vi "vision_webcam_V2.vi"(11 "dup Message Queue 2":refnum<queue>) -> ()   [LabVIEW 2017]
uses:
  UI Error Handlers/support/Message Queue/Message Cluster.ctl
  <vilib>/vision/Image Controls.llb/IMAQ Image.ctl
  camera_array_1.ctl
  <vilib>/userdefined/High Color/IMAQdx.ctl
  <vilib>/vision/Avi.llb/IMAQ AVI2 Refnum.ctl
  <vilib>/vision/Avi.llb/IMAQ AVI2 Codec Path.ctl
  Globals/Global - All RT Loop Stop.vi
  Globals/Global - Configuration Options.vi
  <vilib>/vision/driver/NI_Vision_Acquisition_Software.lvlib
  UI Error Handlers/support/Message Queue/Message Queue.lvlib
panel:
  out "Images":T1
  out "Array":T2[](array[typedef])
  out "Webcam":T2(plugin-control)
  out "Codec Names 2":string[](array[string])
  out "concatenated string 4":string
  out "error out":errorcluster
  out "x-y":u32
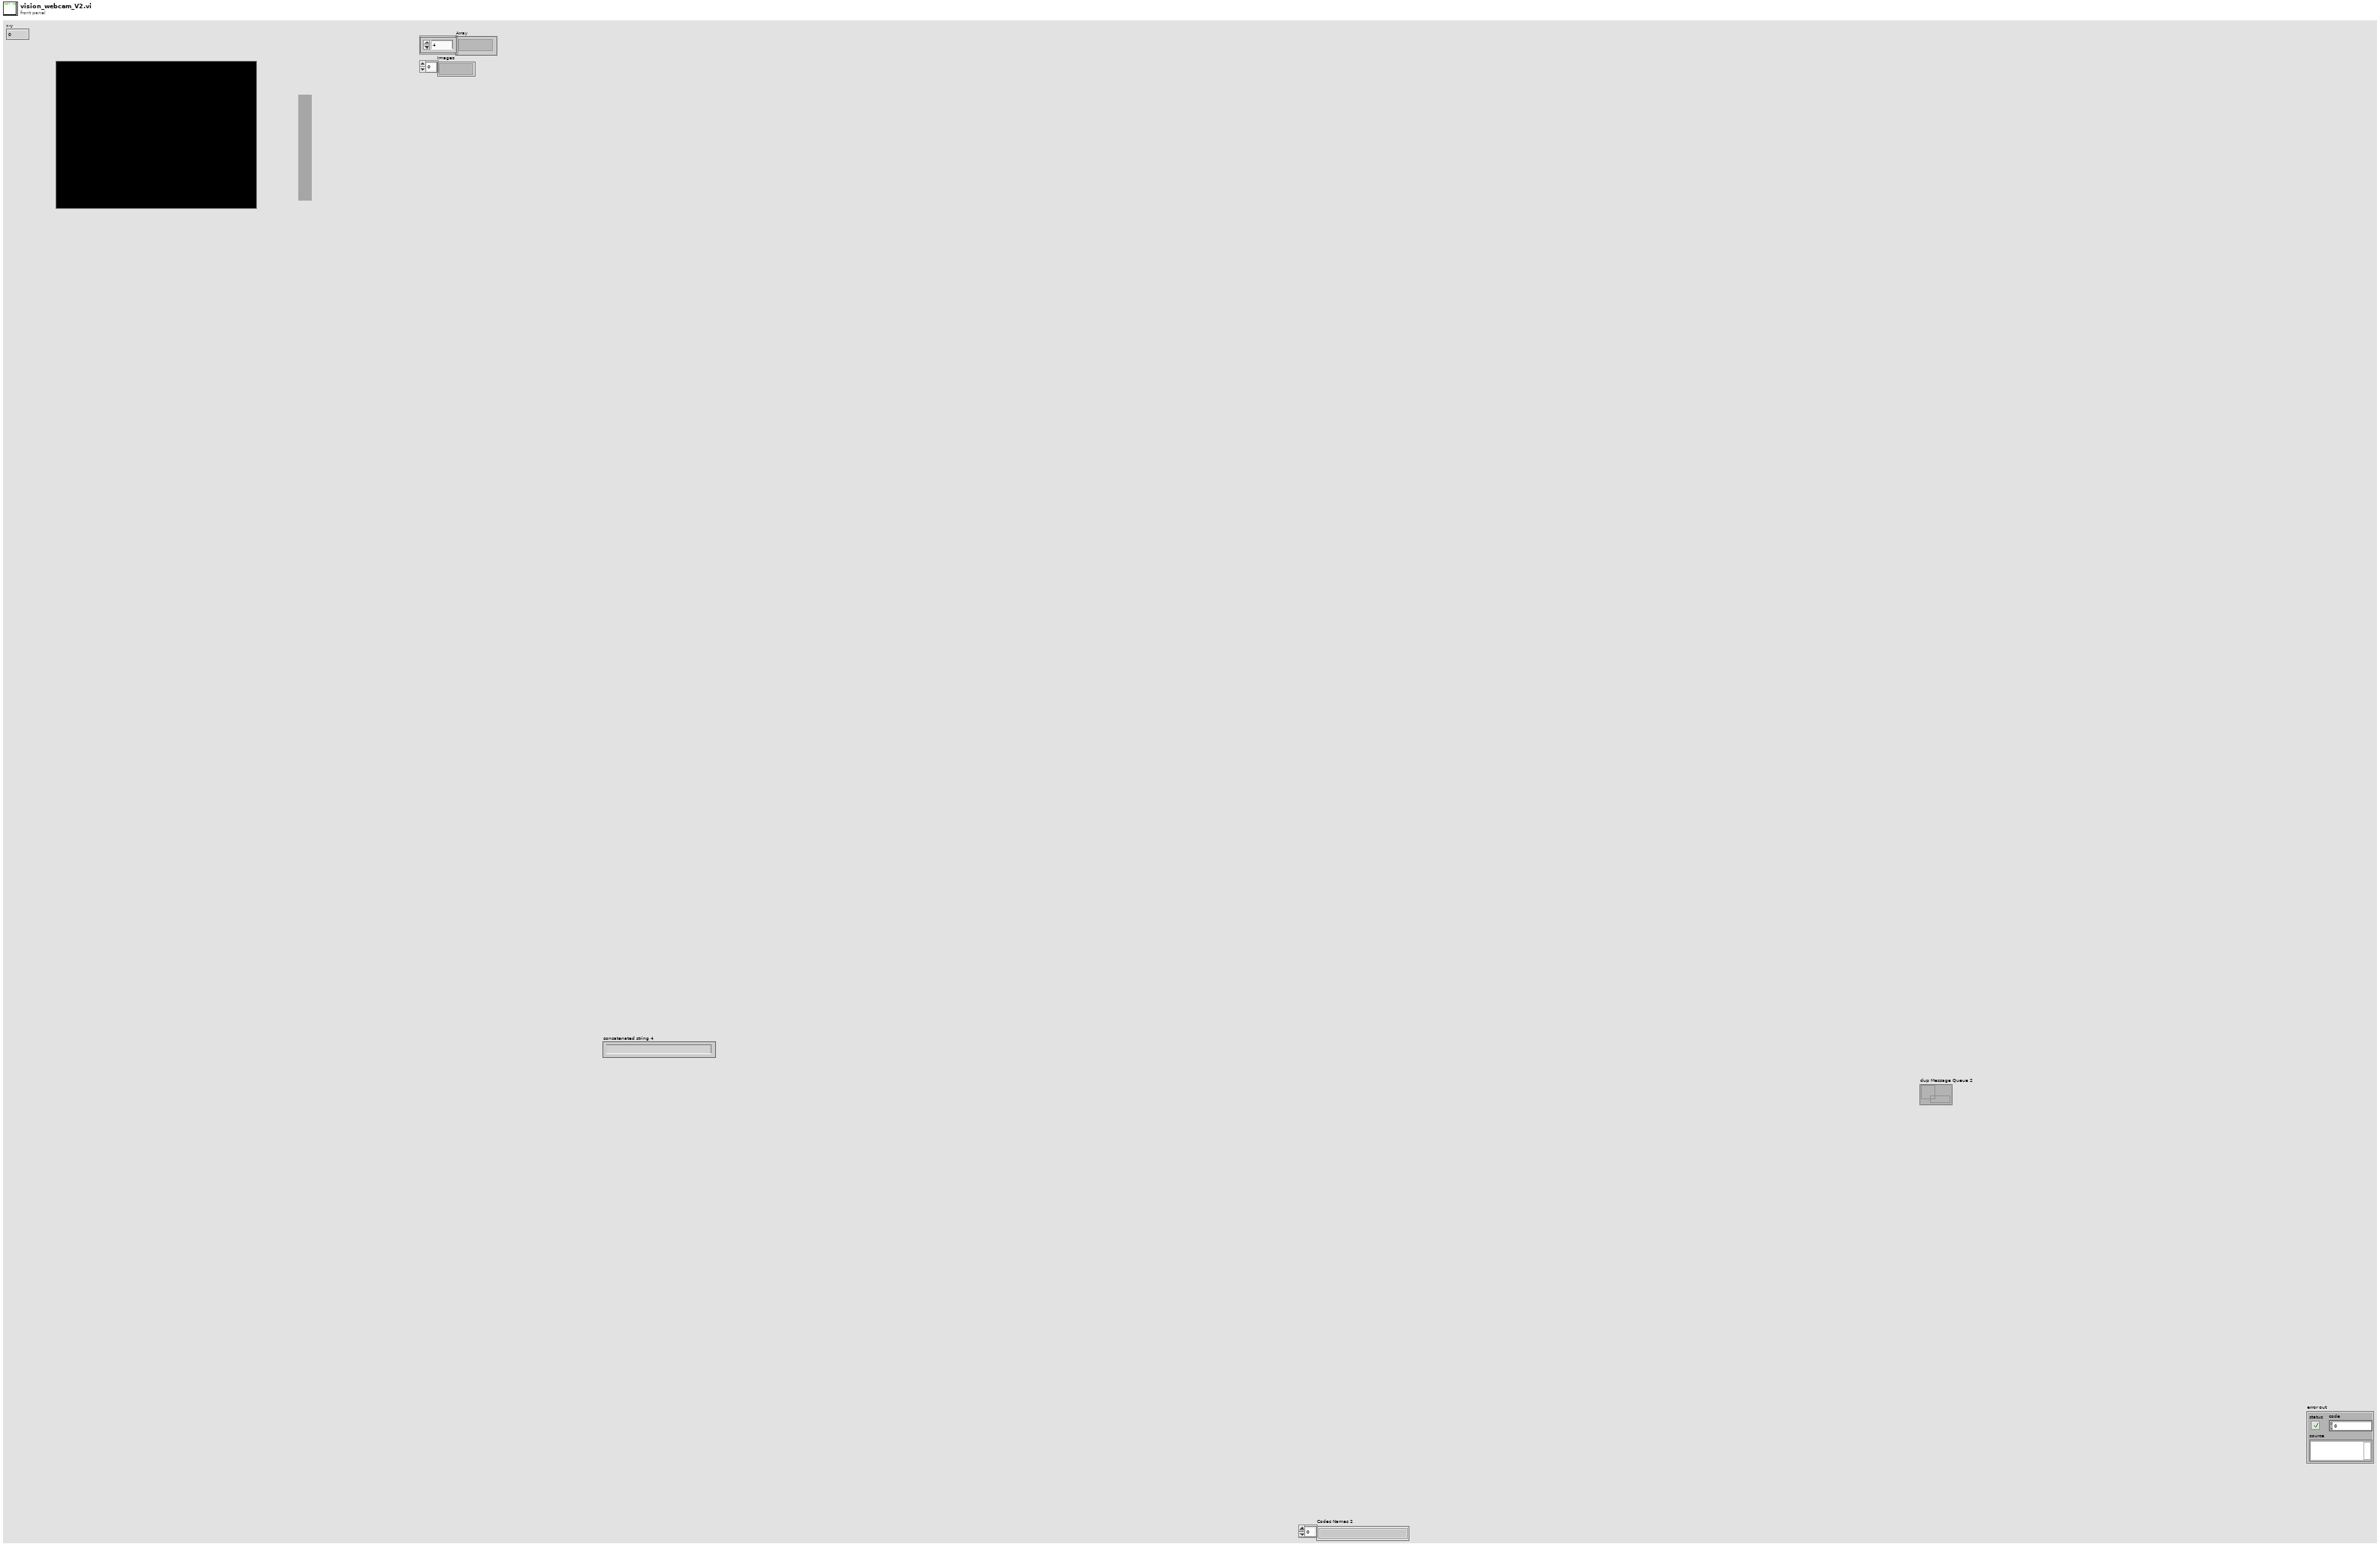
[diagram p1: front panel]
types:
  T1 = typedef "camera_array_1.ctl" = T2[]
  T2 = typedef "IMAQ Image.ctl" = refnum<image>
  T3 = typedef "IMAQ AVI2 Refnum.ctl" = refnum<k20>
  T4 = typedef "IMAQdx.ctl" = refnum<k21>
  T5 = typedef "Image Type" = u32
  T6 = cluster{"Tool data":cluster{"Number of teeth":sgl}, "Cutting data":cluster{"rpm":sgl}, "Limits":cluster{"Magnitude threshold":sgl, "Tolerance":sgl}, "G1 status":cluster{"G1 trigger":bool}}
  T7 = typedef "IMAQ AVI2 Codec Path.ctl" = u32
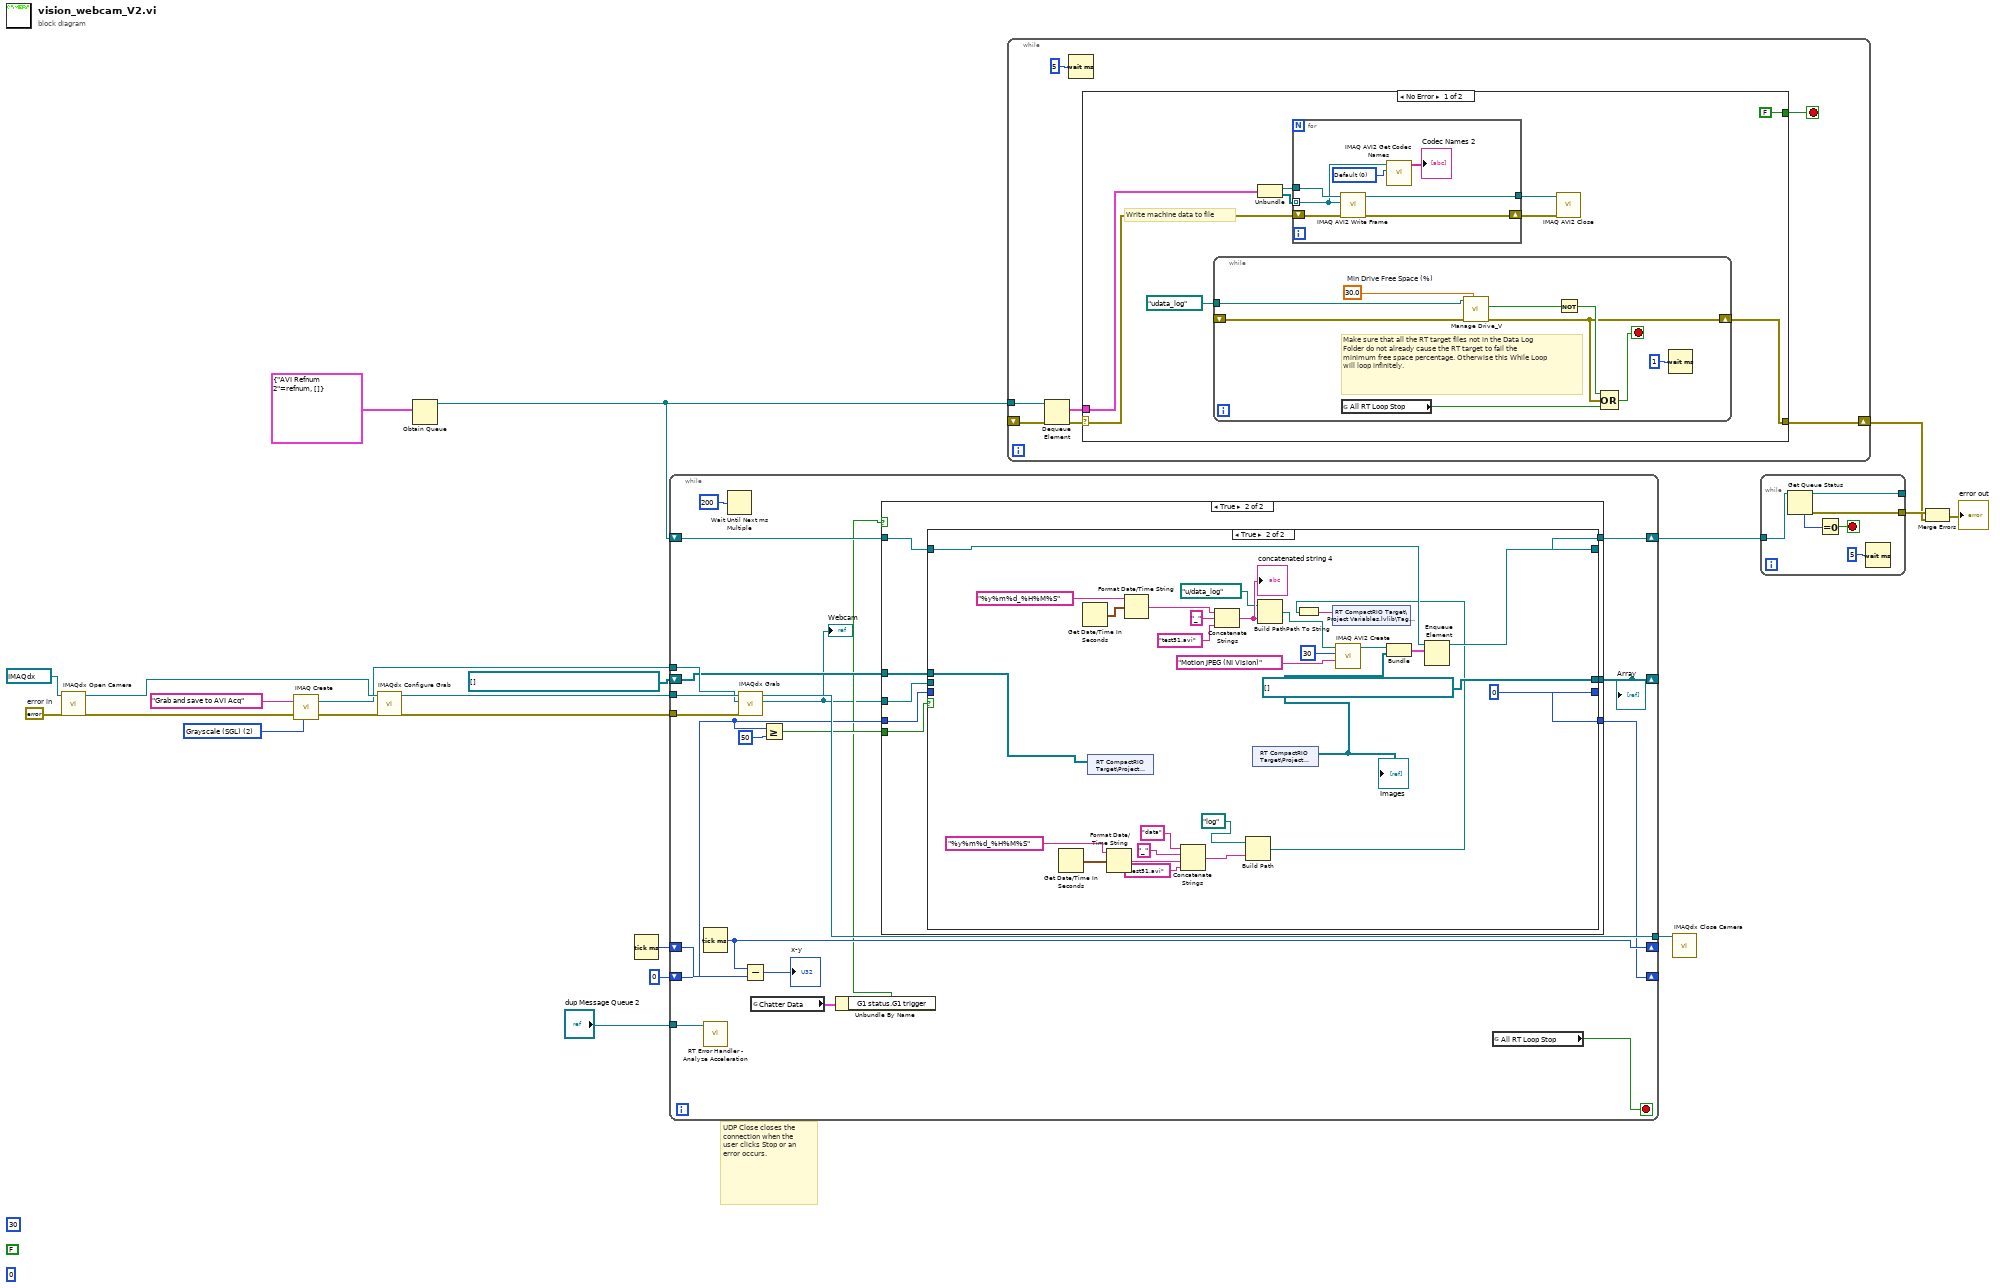
[diagram p0: block diagram]
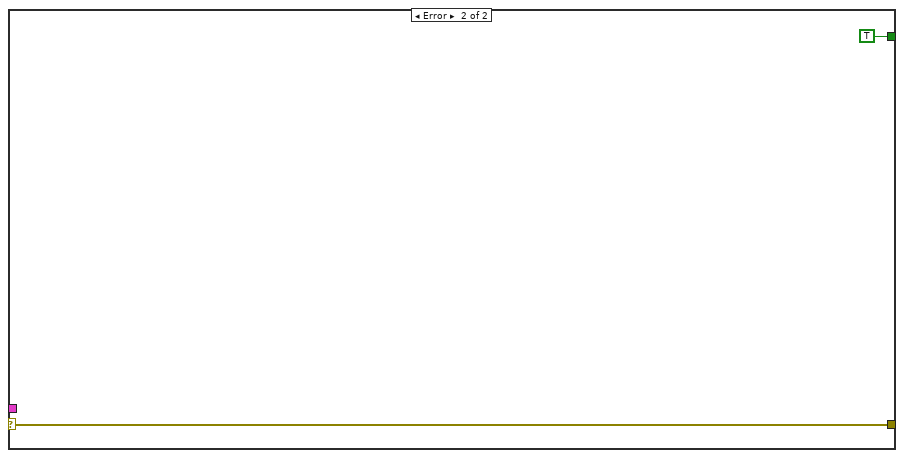
[diagram p2: hidden frame]
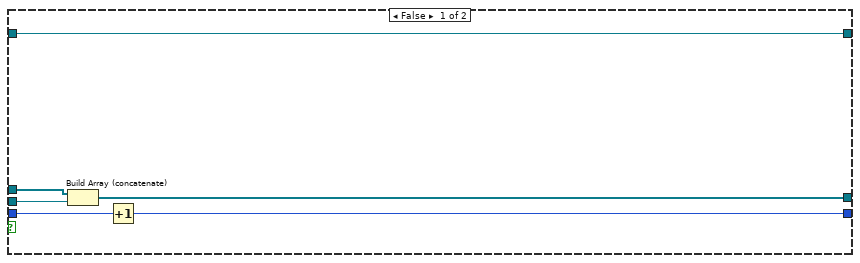
[diagram p4: hidden frame]
diagram:
  w11 = T5 2 items=["Grayscale (U8)", "Grayscale (I16)", "Grayscale (SGL)", "Complex (CSG)", "RGB (U32)", "HSL (U32)", "RGB (U64)", "Grayscale (U16)"] ("Image Type")
  (unwired) u32 30 ("Frames Per Second")
  w12 = errorcluster {"status"=FALSE, "code"=0, "source"=""}  # error in
  (unwired) i16 0 ("A(I16) 11")
  (unwired) FALSE
  # "UDP Close closes the connection when the user clicks Stop or an error occurs."
  n1 = call <vilib>:"IMAQdx Open Camera.vi"("error in"=w12, "Session In"=T4 "cam0") -> ("error out"=w10:errorcluster, "Session Out"=w14:T4)  [unwired: 8 in]
  n2 = call "IMAQ Create"("Image Name"="Grab and save to AVI Acq", "Image Type"=w11, "error in (no error)"=w10) -> ("New Image"=w7:T2, "error out"=w6:errorcluster)  [unwired: 2 in]
  n3 = call <vilib>:"IMAQdx Configure Grab.vi"("error in"=w6, "Session In"=w14) -> ("error out"=w5:errorcluster, "Session Out"=w8:T4)  [unwired: 8 in]
  n4 = Obtain Queue(element data type=cluster{"AVI Refnum 2":T3, T2[]} {"AVI Refnum 2"=refnum, []}) -> (queue out=w19:refnum<queue>)  [unwired: 4 in, 2 out]
  n5 = Tick Count (ms)() -> (millisecond timer value=w15:u32)
  n6 = while {
    shift-right: [w41] -> w21
    shift-left: w19 -> [w42]
    tunnel: "dup Message Queue 2" -> [w40]
    shift-right: [w36] -> _
    shift-left: w15 -> [w37]
    tunnel: w8 -> [w35]
    tunnel: w7 -> [w34]
    tunnel: w5 -> [w33]
    tunnel: [w32] -> w4
    shift-right: [w25] -> _
    shift-left: T2[] [] -> [w29]
    shift-right: [w26] -> _
    shift-left: 0 -> [w27]
    stop <- w24 stop-if-true
    n7 = Tick Count (ms)() -> (millisecond timer value=w36:u32)
    n8 = call "RT Error Handler - Analyze Acceleration.vi"("Message Queue"=w40) -> ()  [unwired: 10 in, 1 out]
    n9 = Wait Until Next ms Multiple(millisecond multiple=u32 200) -> ()  [unwired: 1 out]
    n10 = call <vilib>:"IMAQdx Grab.vi"("error in"=w33, "Image In"=w34, "Session In"=w35) -> ("Image Out"=w22:T2, "Session Out"=w32:T4)  [unwired: 5 in, 2 out]
    "Webcam" <- w22
    n11 = Subtract(x=w36, y=w37) -> (x-y=→"x-y":u32)
    n12 = global read "Global - Configuration Options.vi" "Chatter Data"() -> (w39:T6)
    n13 = Greater Or Equal?(x=w27, y=50) -> (x >= y?=w28:bool)
    n14 = Unbundle By Name(w39) -> ("G1 status.G1 trigger"=w23:bool)
    n15 = case shown="True" w23 {
      tunnel: w42 -> [w45 w46]
      tunnel: [w45 w53] -> w41
      tunnel: w22 -> [_ w52]
      tunnel: w29 -> [w43 w50]
      tunnel: w28 -> [_ w51]
      tunnel: w27 -> [w44 w49]
      tunnel: [w44 w48] -> w26
      tunnel: [w43 w47] -> w25
      frame False {
      }
      frame True {
        n16 = case shown="True" w51 {
          tunnel: [w54 w73] -> w53
          tunnel: w52 -> [w58 _]
          tunnel: w50 -> [w59 w70]
          tunnel: w49 -> [w57 _]
          tunnel: [w56 0] -> w48
          tunnel: [w55 T2[] []] -> w47
          tunnel: w46 -> [w54 w74]
          frame False {
            n17 = Build Array (concatenate)(w59, w58) -> (w55:T2[])
            n18 = Increment(x=w57) -> (x+1=w56:i32)
          }
          frame True {
            n19 = Get Date/Time In Seconds() -> (seconds since 1Jan1904=w67:timestamp)
            n20 = Get Date/Time In Seconds() -> (seconds since 1Jan1904=w84:timestamp)
            n21 = shared-variable "RT CompactRIO Target\\Project Variables.lvlib\\Images"(w70) -> ()  [unwired: 1 in, 1 out]
            n22 = Format Date/Time String(time format string (%c)="%y%m%d_%H%M%S", seconds (now)=w67) -> (date/time string=w66:string)  [unwired: 1 out]
            n23 = Format Date/Time String(time format string (%c)="%y%m%d_%H%M%S", seconds (now)=w84) -> (date/time string=w85:string)  [unwired: 1 out]
            n24 = Concatenate Strings("data" ("string"), "_" ("string"), w66, "test51.avi" ("string")) -> (w68:string)
            n25 = Concatenate Strings(w85, "_" ("string"), "test51.avi" ("name or relative path")) -> (w86:string)
            "concatenated string 4" <- w86
            n26 = Build Path(base path=path "log", name or relative path=w68) -> (appended path=w60:path)
            n27 = shared-variable "RT CompactRIO Target\\Project Variables.lvlib\\Images"() -> (w69:T1)  [unwired: 1 in, 1 out]
            "Images" <- w69
            n28 = Build Path(base path=path "u:/data_log" ("AVI Path"), name or relative path=w86) -> (appended path=w77:path)
            n29 = Path To String(path=w60) -> (string=w87:string)
            n30 = shared-variable "RT CompactRIO Target\\Project Variables.lvlib\\Tag Video"(w87) -> ()  [unwired: 1 in, 1 out]
            n31 = call "IMAQ AVI2 Create"("Codec"="Motion JPEG (NI Vision)", "Frames Per Second"=u32 30, "AVI Path"=w77) -> ("AVI Refnum"=w72:T3)  [unwired: 7 in, 1 out]
            n32 = Bundle("AVI Refnum"=w72, "Array"=w69) -> (w71:cluster{"AVI Refnum":T3, "Array":T1})  [unwired: 1 in]
            n33 = Enqueue Element(queue=w74, element=w71) -> (queue out=w73:refnum<queue>)  [unwired: 2 in, 2 out]
          }
        }
      }
    }
    "Array" <- w25
    n34 = global read "Global - All RT Loop Stop.vi" "All RT Loop Stop"() -> (w24:bool)
  }
  n35 = while {
    tunnel: w19 -> [w94]
    shift-right: [w90] -> w18
    shift-left: _ -> [w93]
    stop <- w91 stop-if-true
    n36 = Dequeue Element(queue=w94, error in (no error)=w93) -> (element=w89:cluster{"AVI Refnum 2":T3, T2[]}, error out=w92:errorcluster)  [unwired: 1 in, 2 out]
    n37 = Wait (ms)(milliseconds to wait=u32 5) -> ()  [unwired: 1 out]
    n38 = case shown="No Error" w92 {
      selector: w92 -> [w102 w120]
      tunnel: [FALSE TRUE] -> w91
      tunnel: [w98 w120] -> w90
      tunnel: w89 -> [w97 _]
      frame No Error {
        # "Write machine data to file"
        n39 = while {
          shift-right: [w114] -> w98
          shift-left: _ -> [w115]
          tunnel: path "/udata_log" ("AVI Path") -> [w112]
          stop <- w119 stop-if-true
          w113 = 30.0  # Min Drive Free Space (%)
          # "Make sure that all the RT target files not in the Data Log Folder do not already cause the RT target to fail the minimum free space percentage. Otherwise this While Loop will loop infinitely."
          n40 = global read "Global - All RT Loop Stop.vi" "All RT Loop Stop"() -> (w116:bool)
          n41 = call "Manage Drive_V.vi"("Min Drive Free Space (%)"=w113, "error in"=w115, "Data Folder"=w112) -> ("error out"=w114:errorcluster, "Drive Space Below Limit"=w111:bool)  [unwired: 6 in, 1 out]
          n42 = Not(x=w111) -> (.not. x?=w118:bool)
          n43 = Compound Arithmetic op=OR(w118, w114, w116) -> (w119:bool)
          n44 = Wait (ms)(milliseconds to wait=u32 1) -> ()  [unwired: 1 out]
        }
        n45 = Unbundle(w97) -> ("AVI Refnum 2"=w96:T3, w95:T2[])
        n46 = for {
          shift-right: [w108] -> w100
          shift-left: w102 -> [w110]
          tunnel: w96 -> [w107]
          tunnel: [w109] -> w101
          tunnel: w95 -> [w104] mode=indexing
          w106 = T7 0 items=["Default", "System", "Built in Vision"] ("Codec Source")
          n47 = call "IMAQ AVI2 Write Frame"("error in (no error)"=w110, "Image"=w104, "AVI Refnum"=w107) -> ("error out"=w108:errorcluster, "AVI Refnum (duplicate)"=w109:T3)  [unwired: 6 in, 1 out]
          n48 = call "IMAQ AVI2 Get Codec Names"("Codec Source"=w106, "Image"=w104) -> ("Codec Names"=→"Codec Names 2":string[])  [unwired: 8 in, 1 out]
        }
        n49 = call "IMAQ AVI2 Close"("error in (no error)"=w100, "AVI Refnum"=w101) -> ()  [unwired: 9 in, 1 out]
      }
      frame Error {
      }
    }
  }
  n50 = call <vilib>:"IMAQdx Close Camera.vi"("Session In"=w4) -> ()  [unwired: 10 in, 1 out]
  n51 = while {
    tunnel: [w126] -> w20
    tunnel: [w124] -> _
    tunnel: w21 -> [w122]
    stop <- w125 stop-if-true
    n52 = Get Queue Status(queue=w122) -> (queue out=w124:refnum<queue>, error out=w126:errorcluster, # elements in queue=w123:i32)  [unwired: 2 in, 5 out]
    n53 = Equal To 0?(x=w123) -> (x = 0?=w125:bool)
    n54 = Wait (ms)(milliseconds to wait=u32 5) -> ()  [unwired: 1 out]
  }
  n55 = Merge Errors(w20, w18) -> (→"error out":errorcluster)
